vi "D1 (1).vi"() -> ()   [LabVIEW 2020]
panel:
  in  "Right":bool
  in  "Left":bool
  in  "Down":bool
  in  "Up":bool
  in  "Exit":bool
  out "Score":dbl
  in  "New Game":bool
  in  "Lost":string
  in  "Won":string
  in  "Colors":u32[](array[colorbox])=[12369084, 13881005, 10130036, 16761177, 16736768, 11814144, 14419712, 13469951, 4991743, 4376575, 8978358, 3126272]
  in  "Board":i32[][](array[numeric])=[[0, 0, 0, 0], [0, 0, 0, 0], [0, 0, 0, 0], [0, 0, 0, 0]]
  out "Tiles":refnum<vi>[][](array[refnum])
  in  "Title 16":bool
  in  "Title 15":bool
  in  "Title 14":bool
  in  "Title 13":bool
  in  "Title 12":bool
  in  "Title 11":bool
  in  "Title 10":bool
  in  "Title 9":bool
  in  "Title 8":bool
  in  "Title 7":bool
  in  "Title 6":bool
  in  "Title 5":bool
  in  "Title 4":bool
  in  "Title 3":bool
  in  "Title 2":bool
  in  "Title 1":bool
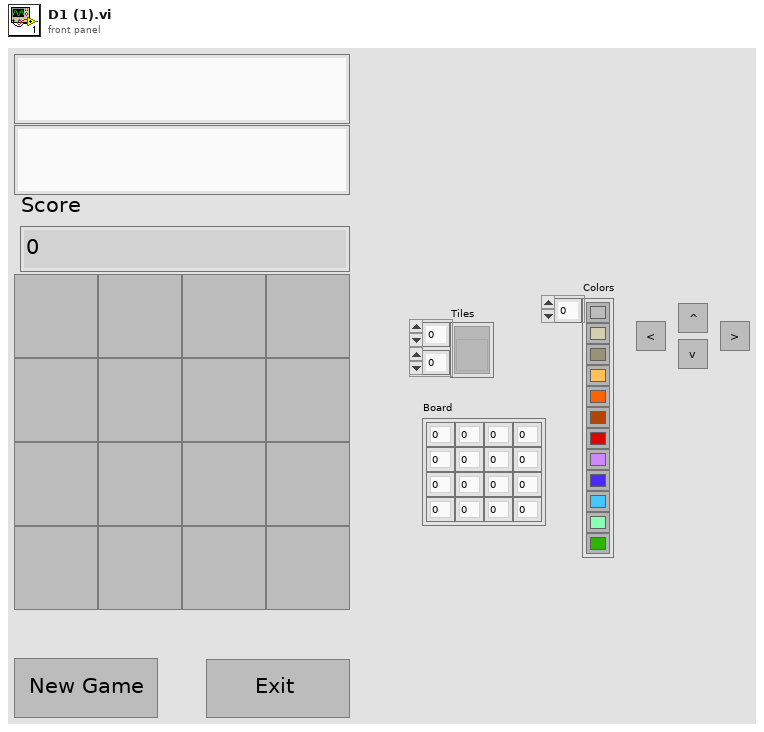
[diagram p1: front panel]
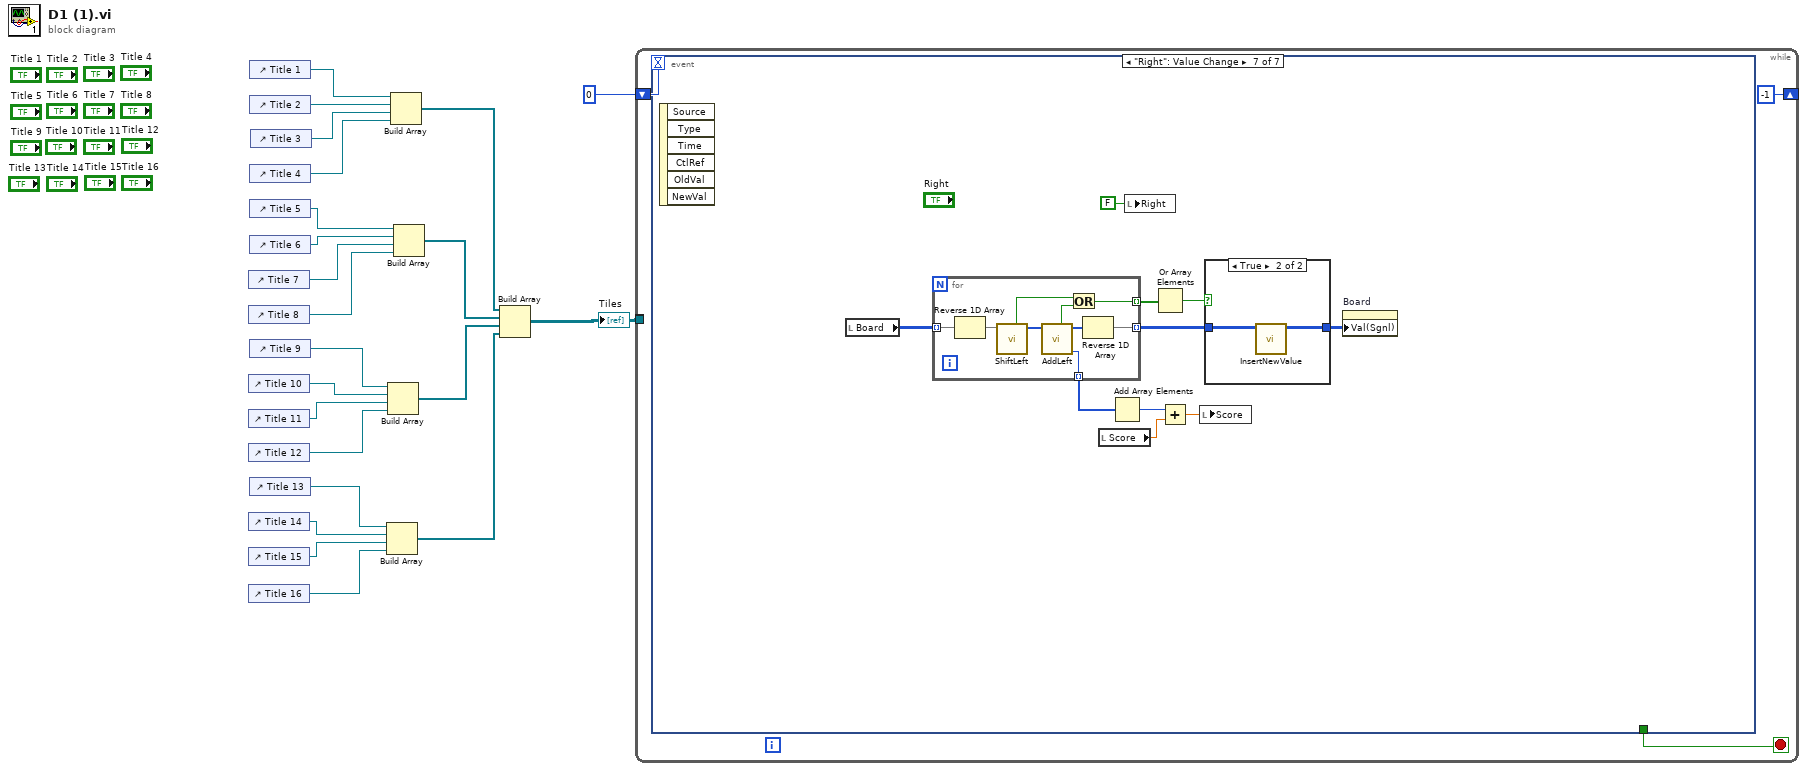
[diagram p0: block diagram]
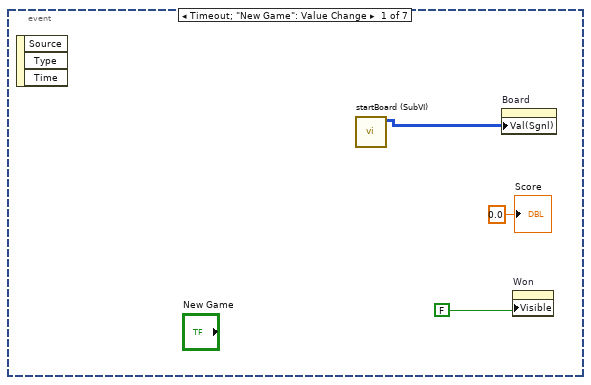
[diagram p2: hidden frame]
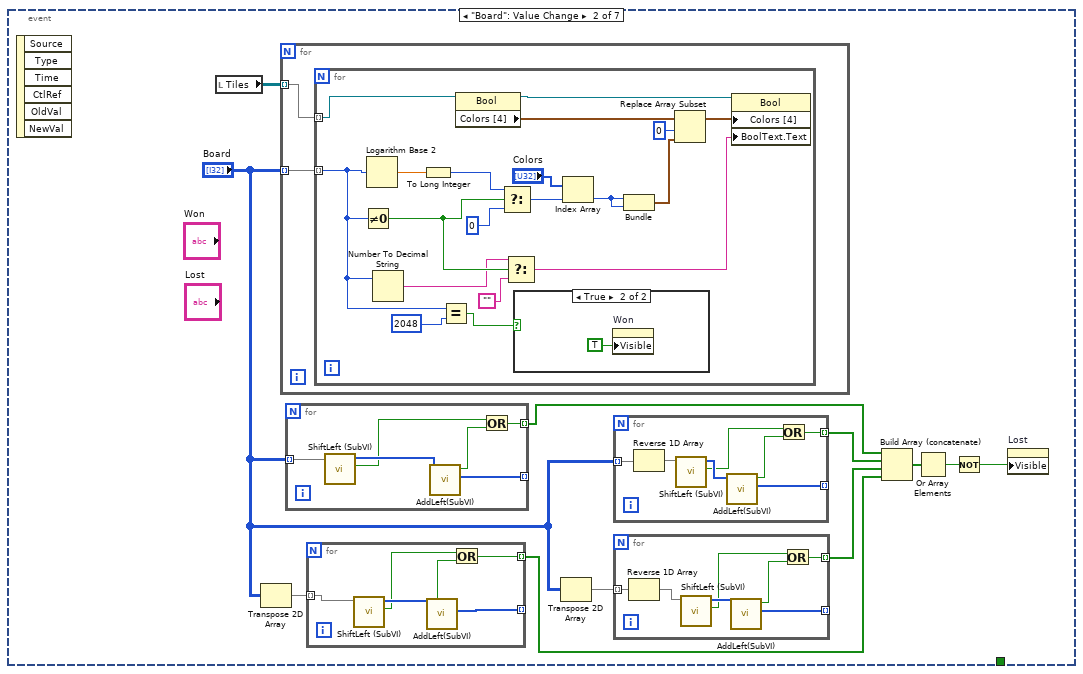
[diagram p3: hidden frame]
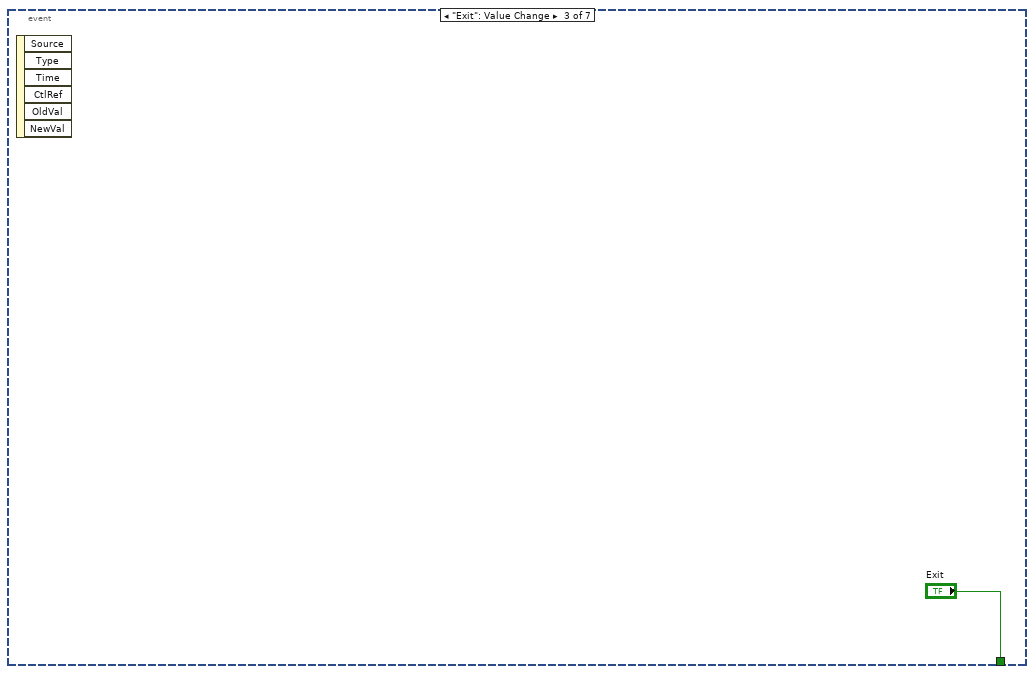
[diagram p5: hidden frame]
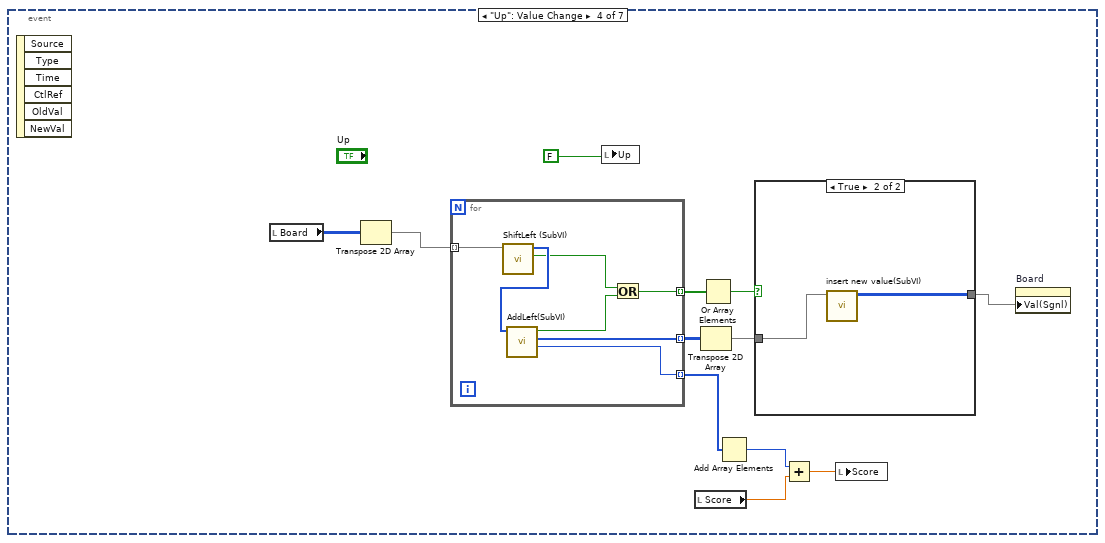
[diagram p6: hidden frame]
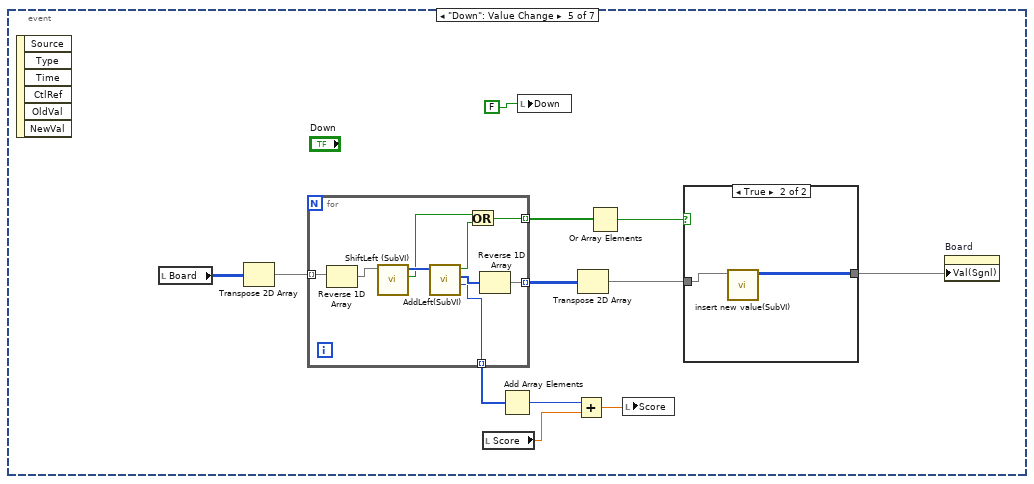
[diagram p8: hidden frame]
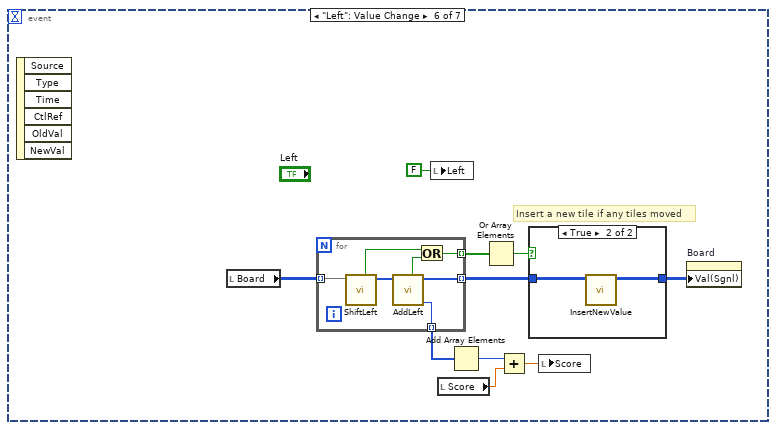
[diagram p10: hidden frame]
diagram:
  n1 = control-ref of="Title 7"() -> (w11:refnum<vi>)
  n2 = control-ref of="Title 8"() -> (w10:refnum<vi>)
  n3 = control-ref of="Title 10"() -> (w8:refnum<vi>)
  n4 = control-ref of="Title 11"() -> (w7:refnum<vi>)
  n5 = control-ref of="Title 12"() -> (w6:refnum<vi>)
  n6 = control-ref of="Title 14"() -> (w4:refnum<vi>)
  n7 = control-ref of="Title 15"() -> (w3:refnum<vi>)
  n8 = control-ref of="Title 16"() -> (w2:refnum<vi>)
  n9 = control-ref of="Title 1"() -> (w17:refnum<vi>)
  n10 = control-ref of="Title 2"() -> (w16:refnum<vi>)
  n11 = control-ref of="Title 4"() -> (w14:refnum<vi>)
  n12 = control-ref of="Title 5"() -> (w13:refnum<vi>)
  n13 = control-ref of="Title 6"() -> (w12:refnum<vi>)
  n14 = control-ref of="Title 9"() -> (w9:refnum<vi>)
  n15 = control-ref of="Title 13"() -> (w5:refnum<vi>)
  n16 = control-ref of="Title 3"() -> (w15:refnum<vi>)
  n17 = Build Array(w5, w4, w3, w2) -> (w18:refnum<vi>[])
  n18 = Build Array(w9, w8, w7, w6) -> (w21:refnum<vi>[])
  n19 = Build Array(w17, w16, w15, w14) -> (w19:refnum<vi>[])
  n20 = Build Array(w13, w12, w11, w10) -> (w20:refnum<vi>[])
  n21 = Build Array(w19, w20, w21, w18) -> (w1:refnum<vi>[][])
  "Tiles" <- w1
  n22 = while {
    tunnel: [w26] -> _
    tunnel: w1 -> [w26]
    shift-right: [-1] -> _
    shift-left: 0 -> [w24]
    stop <- w23 stop-if-true
    n23 = event shown="[6] \"Right\": Value Change" {
      selector: _ -> [_ _ _ _ _ _ _]
      dyn-events: _ -> [_ _ _ _ _ _ _]
      timeout: w24 -> [_ _ _ _ _ _ _]
      tunnel: [_ _ "Exit" _ _ _ _] -> w23
      event Timeout; "New Game": Value Change {
        n24 = event-data() -> ()  [unwired: 1 in, 3 out]
        n25 = call "startBoard (SubVI).vi"() -> ("output array"=w29:i32[][])  [unwired: 11 in]
        n26 = property on="Board" class="Arr (strict)"("Val(Sgnl)"=w29) -> ()  [unwired: 2 in, 2 out]
        n27 = property on="Won" class="Str"("Visible"=FALSE) -> ()  [unwired: 2 in, 2 out]
        "Score" <- 0.0 ("Score")
      }
      event "Board": Value Change {
        n28 = event-data() -> ()  [unwired: 1 in, 6 out]
        n29 = local read "Tiles"() -> (w40:refnum<vi>[][])
        n30 = Transpose 2D Array(2D array="Board") -> (transposed array=w39:i32[][])
        n31 = for {
          tunnel: w40 -> [w68] mode=indexing
          tunnel: "Board" -> [w67] mode=indexing
          n32 = for {
            tunnel: w68 -> [w77] mode=indexing
            tunnel: w67 -> [w81] mode=indexing
            n33 = Not Equal To 0?(x=w81) -> (x != 0?=w84:bool)
            n34 = Logarithm Base 2(1:w81) -> (0:w87:dbl)
            n35 = Number To Decimal String(number=w81) -> (decimal integer string=w83:string)  [unwired: 1 in]
            n36 = To Long Integer(number=w87) -> (32bit integer=w86:i32)
            n37 = Equal?(x=w81, y=2048) -> (x = y?=w79:bool)
            n38 = property class="Bool"(reference=w77) -> (reference out=w71:refnum<vi>, "Colors [4]"=w74:cluster{u32, u32}[])  [unwired: 1 in, 1 out]
            n39 = Select(t=w86, s=w84, f=0) -> (s? t:f=w78:i32)
            n40 = Select(t=w83, s=w84, f="") -> (s? t:f=w69:string)
            n41 = case shown="True" w79 {
              frame False {
              }
              frame True {
                n42 = property on="Won" class="Str"("Visible"=TRUE) -> ()  [unwired: 2 in, 2 out]
              }
            }
            n43 = Index Array(array="Colors", index=w78) -> (element=w75:u32)
            n44 = Bundle("Color Box 2"=w75, "Color Box 2"=w75) -> (w73:cluster{"Color Box 2":u32, "Color Box 2":u32})  [unwired: 1 in]
            n45 = Replace Array Subset(array=w74, new element=w73, index=0) -> (w70:cluster{u32, u32}[])
            n46 = property class="Bool"(reference=w71, "Colors [4]"=w70, "BoolText.Text"=w69) -> ()  [unwired: 1 in, 2 out]
          }
        }
        n47 = for {
          tunnel: "Board" -> [w61] mode=indexing
          tunnel: [w66] -> w36 mode=indexing
          tunnel: [w64] -> _ mode=indexing
          n48 = call "ShiftLeft (SubVI).vi"("Array in"=w61) -> ("tiles moved?"=w62:bool, "Array out"=w63:i32[])  [unwired: 9 in]
          n49 = call "AddLeft(SubVI).vi"("Array in"=w63) -> ("Array out"=w64:i32[], "tiles moved?"=w65:bool)  [unwired: 8 in, 1 out]
          n50 = Or(x=w62, y=w65) -> (x .or. y?=w66:bool)
        }
        n51 = for {
          tunnel: [w59] -> _ mode=indexing
          tunnel: [w58] -> w35 mode=indexing
          tunnel: w39 -> [w57] mode=indexing
          n52 = call "ShiftLeft (SubVI).vi"("Array in"=w57) -> ("tiles moved?"=w55:bool, "Array out"=w56:i32[])  [unwired: 9 in]
          n53 = call "AddLeft(SubVI).vi"("Array in"=w56) -> ("Array out"=w59:i32[], "tiles moved?"=w60:bool)  [unwired: 8 in, 1 out]
          n54 = Or(x=w55, y=w60) -> (x .or. y?=w58:bool)
        }
        n55 = Transpose 2D Array(2D array="Board") -> (transposed array=w37:i32[][])
        n56 = for {
          tunnel: "Board" -> [w51] mode=indexing
          tunnel: [w53] -> w33 mode=indexing
          tunnel: [w52] -> _ mode=indexing
          n57 = Reverse 1D Array(array=w51) -> (reversed array=w50:i32[])
          n58 = call "ShiftLeft (SubVI).vi"("Array in"=w50) -> ("tiles moved?"=w48:bool, "Array out"=w49:i32[])  [unwired: 9 in]
          n59 = call "AddLeft(SubVI).vi"("Array in"=w49) -> ("Array out"=w52:i32[], "tiles moved?"=w54:bool)  [unwired: 8 in, 1 out]
          n60 = Or(x=w48, y=w54) -> (x .or. y?=w53:bool)
        }
        n61 = for {
          tunnel: [w46] -> w34 mode=indexing
          tunnel: [w45] -> _ mode=indexing
          tunnel: w37 -> [w44] mode=indexing
          n62 = Reverse 1D Array(array=w44) -> (reversed array=w43:i32[])
          n63 = call "ShiftLeft (SubVI).vi"("Array in"=w43) -> ("tiles moved?"=w41:bool, "Array out"=w42:i32[])  [unwired: 9 in]
          n64 = call "AddLeft(SubVI).vi"("Array in"=w42) -> ("Array out"=w45:i32[], "tiles moved?"=w47:bool)  [unwired: 8 in, 1 out]
          n65 = Or(x=w41, y=w47) -> (x .or. y?=w46:bool)
        }
        n66 = Build Array (concatenate)(w36, w33, w34, w35) -> (w32:bool[])
        n67 = Or Array Elements(Boolean array=w32) -> (logical OR=w31:bool)
        n68 = Not(x=w31) -> (.not. x?=w30:bool)
        n69 = property on="Lost" class="Str"("Visible"=w30) -> ()  [unwired: 2 in, 2 out]
      }
      event "Exit": Value Change {
        n70 = event-data() -> ()  [unwired: 1 in, 6 out]
      }
      event "Up": Value Change {
        n71 = event-data() -> ()  [unwired: 1 in, 6 out]
        n72 = local read "Board"() -> (w100:i32[][])
        n73 = Transpose 2D Array(2D array=w100) -> (transposed array=w99:i32[][])
        n74 = for {
          tunnel: w99 -> [w110] mode=indexing
          tunnel: [w107] -> w98 mode=indexing
          tunnel: [w106] -> w97 mode=indexing
          tunnel: [w105] -> w93 mode=indexing
          n75 = call "ShiftLeft (SubVI).vi"("Array in"=w110) -> ("tiles moved?"=w109:bool, "Array out"=w111:i32[])  [unwired: 9 in]
          n76 = call "AddLeft(SubVI).vi"("Array in"=w111) -> ("Score"=w105:i32, "Array out"=w106:i32[], "tiles moved?"=w108:bool)  [unwired: 8 in]
          n77 = Or(x=w109, y=w108) -> (x .or. y?=w107:bool)
        }
        n78 = local write "Up"(FALSE) -> ()
        n79 = local read "Score"() -> (w91:dbl)
        n80 = Transpose 2D Array(2D array=w97) -> (transposed array=w95:i32[][])
        n81 = Or Array Elements(Boolean array=w98) -> (logical OR=w96:bool)
        n82 = Add Array Elements(numeric array=w93) -> (sum=w92:i32)
        n83 = case shown="True" w96 {
          tunnel: w95 -> [w102 w104]
          tunnel: [w102 w103] -> w94
          frame False {
          }
          frame True {
            n84 = call "insert new value(SubVI).vi"("Board"=w104) -> ("output"=w103:i32[][])  [unwired: 10 in]
          }
        }
        n85 = Add(x=w92, y=w91) -> (x+y=w90:dbl)
        n86 = local write "Score"(w90) -> ()
        n87 = property on="Board" class="Arr (strict)"("Val(Sgnl)"=w94) -> ()  [unwired: 2 in, 2 out]
      }
      event "Down": Value Change {
        n88 = event-data() -> ()  [unwired: 1 in, 6 out]
        n89 = local read "Board"() -> (w122:i32[][])
        n90 = Transpose 2D Array(2D array=w122) -> (transposed array=w123:i32[][])
        n91 = for {
          tunnel: [w133] -> w113 mode=indexing
          tunnel: [w129] -> w116 mode=indexing
          tunnel: [w128] -> w120 mode=indexing
          tunnel: w123 -> [w127] mode=indexing
          n92 = Reverse 1D Array(array=w127) -> (reversed array=w135:i32[])
          n93 = call "ShiftLeft (SubVI).vi"("Array in"=w135) -> ("tiles moved?"=w131:bool, "Array out"=w134:i32[])  [unwired: 9 in]
          n94 = call "AddLeft(SubVI).vi"("Array in"=w134) -> ("Score"=w128:i32, "Array out"=w130:i32[], "tiles moved?"=w132:bool)  [unwired: 8 in]
          n95 = Or(x=w131, y=w132) -> (x .or. y?=w133:bool)
          n96 = Reverse 1D Array(array=w130) -> (reversed array=w129:i32[])
        }
        n97 = local read "Score"() -> (w118:dbl)
        n98 = Add Array Elements(numeric array=w120) -> (sum=w119:i32)
        n99 = local write "Down"(FALSE) -> ()
        n100 = Add(x=w119, y=w118) -> (x+y=w117:dbl)
        n101 = Transpose 2D Array(2D array=w116) -> (transposed array=w115:i32[][])
        n102 = Or Array Elements(Boolean array=w113) -> (logical OR=w114:bool)
        n103 = local write "Score"(w117) -> ()
        n104 = case shown="True" w114 {
          tunnel: w115 -> [w124 w126]
          tunnel: [w124 w125] -> w112
          frame False {
          }
          frame True {
            n105 = call "insert new value(SubVI).vi"("Board"=w126) -> ("output"=w125:i32[][])  [unwired: 10 in]
          }
        }
        n106 = property on="Board" class="Arr (strict)"("Val(Sgnl)"=w112) -> ()  [unwired: 2 in, 2 out]
      }
      event "Left": Value Change {
        # "Insert a new tile if any tiles moved"
        n107 = event-data() -> ()  [unwired: 1 in, 6 out]
        n108 = local read "Board"() -> (w144:i32[][])
        n109 = for {
          tunnel: w144 -> [w155] mode=indexing
          tunnel: [w153] -> w143 mode=indexing
          tunnel: [w152] -> w139 mode=indexing
          tunnel: [w149] -> w137 mode=indexing
          n110 = call "ShiftLeft.vi"("Array"=w155) -> ("Array 2"=w154:i32[], "tiles moved?"=w150:bool)  [unwired: 9 in]
          n111 = call "AddLeft.vi"("Array"=w154) -> ("score"=w152:i32, "Array 2"=w153:i32[], "tiles moved?"=w151:bool)  [unwired: 8 in]
          n112 = Or(x=w150, y=w151) -> (x .or. y?=w149:bool)
        }
        n113 = local write "Left"(FALSE ("Left")) -> ()
        n114 = local read "Score"() -> (w140:dbl)
        n115 = Add Array Elements(numeric array=w139) -> (sum=w142:i32)
        n116 = Or Array Elements(Boolean array=w137) -> (logical OR=w136:bool)
        n117 = Add(x=w142, y=w140) -> (x+y=w141:dbl)
        n118 = case shown="True" w136 {
          tunnel: w143 -> [w146 w148]
          tunnel: [w146 w147] -> w138
          frame False {
          }
          frame True {
            n119 = call "InsertNewValue.vi"("Board"=w148) -> ("output"=w147:i32[][])  [unwired: 10 in]
          }
        }
        n120 = local write "Score"(w141) -> ()
        n121 = property on="Board" class="Arr (strict)"("Val(Sgnl)"=w138) -> ()  [unwired: 2 in, 2 out]
      }
      event "Right": Value Change {
        n122 = event-data() -> ()  [unwired: 1 in, 6 out]
        n123 = local read "Board"() -> (w164:i32[][])
        n124 = for {
          tunnel: w164 -> [w175] mode=indexing
          tunnel: [w173] -> w163 mode=indexing
          tunnel: [w172] -> w159 mode=indexing
          tunnel: [w169] -> w157 mode=indexing
          n125 = Reverse 1D Array(array=w175) -> (reversed array=w174:i32[])
          n126 = call "ShiftLeft.vi"("Array"=w174) -> ("Array 2"=w177:i32[], "tiles moved?"=w170:bool)  [unwired: 9 in]
          n127 = call "AddLeft.vi"("Array"=w177) -> ("score"=w172:i32, "Array 2"=w176:i32[], "tiles moved?"=w171:bool)  [unwired: 8 in]
          n128 = Or(x=w170, y=w171) -> (x .or. y?=w169:bool)
          n129 = Reverse 1D Array(array=w176) -> (reversed array=w173:i32[])
        }
        n130 = local read "Score"() -> (w160:dbl)
        n131 = Add Array Elements(numeric array=w159) -> (sum=w162:i32)
        n132 = local write "Right"(FALSE ("Right")) -> ()
        n133 = Or Array Elements(Boolean array=w157) -> (logical OR=w156:bool)
        n134 = Add(x=w162, y=w160) -> (x+y=w161:dbl)
        n135 = local write "Score"(w161) -> ()
        n136 = case shown="True" w156 {
          tunnel: w163 -> [w166 w168]
          tunnel: [w166 w167] -> w158
          frame False {
          }
          frame True {
            n137 = call "InsertNewValue.vi"("Board"=w168) -> ("output"=w167:i32[][])  [unwired: 10 in]
          }
        }
        n138 = property on="Board" class="Arr (strict)"("Val(Sgnl)"=w158) -> ()  [unwired: 2 in, 2 out]
      }
    }
  }
